vi "CRYDelete DataView Array Idx.vi"(11 "DataView Idx In":i32) -> ()   [LabVIEW 2013]
uses:
  CRYNew View Global.vi
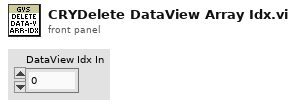
[diagram p1: front panel]
types:
  T1 = typedef "Graph Main Info Cluster.ctl" = cluster{"Selected_BarIdx":i32, "Selected_PanelIdx":i32, "Graph Main VIRef":refnum<vi>, "ToolBarClick":bool, "Spliter Ref Array":refnum<vi>[], "Panel Ref Array":refnum<vi>[], "Spliter_matrix":i32[][], "Panel_matrix":i32[][], "child_spliterIdx_matrix":i32[][], "split_pos_matrix":i32[][], "Title State":bool, "sQueueName":string, "Frame nID":i32, "Graph VIRef Array":cluster{"Graph VIRef":refnum<vi>, "Panel Idx":i32, "Frame VIRef":refnum<vi>, "Icon Ring":i32, "Graph Type":string}[], "View Type":string}
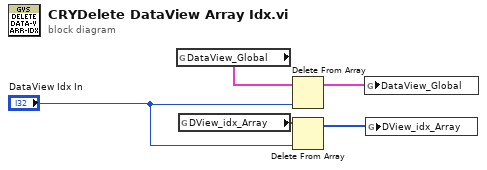
[diagram p0: block diagram]
diagram:
  n1 = global read "CRYNew View Global.vi" "DataView_Global"() -> (w5:T1[])
  n2 = global read "CRYNew View Global.vi" "DView_idx_Array"() -> (w4:i32[])
  n3 = Delete From Array(array=w5, index="DataView Idx In") -> (array with subset deleted=w3:T1[])  [unwired: 1 in, 1 out]
  n4 = Delete From Array(array=w4, index="DataView Idx In") -> (array with subset deleted=w2:i32[])  [unwired: 1 in, 1 out]
  n5 = global write "CRYNew View Global.vi" "DataView_Global"(w3) -> ()
  n6 = global write "CRYNew View Global.vi" "DView_idx_Array"(w2) -> ()
